vi "Sort into Arrival Time Buffer.vi"(5 "Time Low":u32[][](array[numeric]), 6 "Delay, ns":u32, 7 "Time High":u32[][](array[numeric]), 8 "Channel buffers are synchronized":bool, 9 "Size of Channel Arrays":u32[](array[numeric]), 10 "Buffer In":i32[][](array[numeric]), 11 "Number of Photons Counted In":i32) -> (1 "Index for Buffer":i32[](array[numeric]), 2 "Buffer Out":i32[][](array[numeric]), 3 "Number of Photons Counted Out":i32)   [LabVIEW 2009]
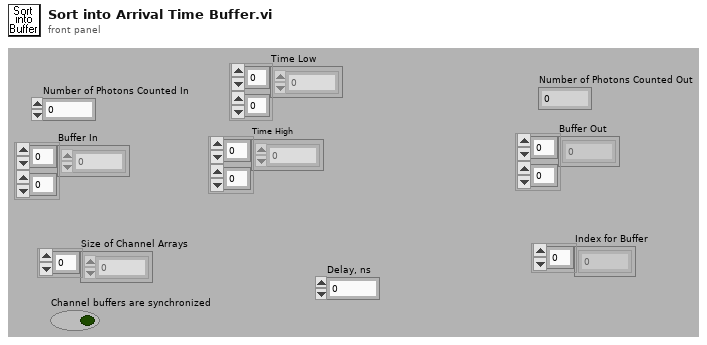
[diagram p1: front panel]
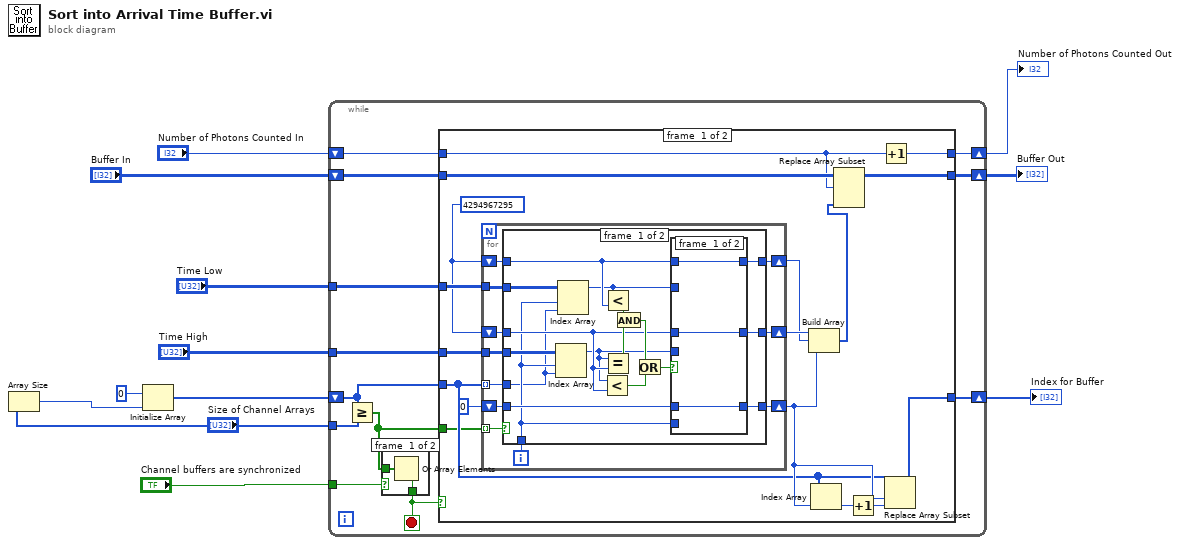
[diagram p0: block diagram]
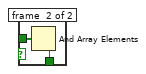
[diagram p2: hidden frame]
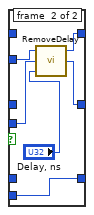
[diagram p3: hidden frame]
diagram:
  n1 = Array Size(array="Size of Channel Arrays") -> (size(s)=w1:i32)
  n2 = Initialize Array(0 ("Element Data"), w1) -> (w5:i32[])
  n3 = while {
    tunnel: "Channel buffers are synchronized" -> [w13]
    shift-left: "Number of Photons Counted In" -> [w18]
    shift-right: [w17] -> w12
    shift-left: "Buffer In" -> [w22]
    shift-right: [w19] -> w8
    shift-left: w5 -> [w23]
    shift-right: [w16] -> w10
    tunnel: "Size of Channel Arrays" -> [w24]
    tunnel: "Time High" -> [w20]
    tunnel: "Time Low" -> [w21]
    stop <- w14 stop-if-true
    n4 = Greater Or Equal?(x=w23, y=w24) -> (x >= y?=w15:bool[])
    n5 = case shown="True" w13 {
      tunnel: [w26 w27] -> w14
      tunnel: w15 -> [w25 w28]
      frame #0 {
        n6 = Or Array Elements(Boolean array=w25) -> (logical OR=w26:bool)
      }
      frame #1 {
        n7 = And Array Elements(Boolean array=w28) -> (logical AND=w27:bool)
      }
    }
    n8 = case shown="False" w14 {
      tunnel: w23 -> [w32 w86]
      tunnel: w22 -> [w41 w88]
      tunnel: w21 -> [w45 _]
      tunnel: w20 -> [w44 _]
      tunnel: [w40 w88] -> w19
      tunnel: [w38 w87] -> w17
      tunnel: w18 -> [w39 w87]
      tunnel: [w31 w86] -> w16
      tunnel: w15 -> [w30 _]
      frame #0 {
        w43 = u32 4294967295
        n9 = for {
          tunnel: w45 -> [w56]
          tunnel: w44 -> [w55]
          tunnel: w32 -> [w53] mode=indexing
          shift-right: [w49] -> w36
          shift-left: w43 -> [w51]
          shift-right: [w48] -> w37
          shift-left: w43 -> [w52]
          shift-right: [w47] -> w33
          shift-left: 0 -> [w50]
          tunnel: w30 -> [w46] mode=indexing
          i -> [w54]
          n10 = case shown="False" w46 {
            tunnel: w56 -> [w62 _]
            tunnel: w55 -> [w60 _]
            tunnel: w54 -> [w59 _]
            tunnel: w53 -> [w58 _]
            tunnel: w52 -> [w68 w84]
            tunnel: w51 -> [w67 w85]
            tunnel: w50 -> [w66 w83]
            tunnel: [w65 w85] -> w49
            tunnel: [w64 w84] -> w48
            tunnel: [w63 w83] -> w47
            frame #0 {
              n11 = Index Array(array=w60, index (row)=w59, index (col)=w58) -> (element=w57:u32)
              n12 = Index Array(array=w62, index (row)=w59, index (col)=w58) -> (element=w61:u32)
              n13 = Less?(x=w57, y=w68) -> (x < y?=w71:bool)
              n14 = Less?(x=w61, y=w67) -> (x < y?=w73:bool)
              n15 = Equal?(x=w57, y=w68) -> (x = y?=w72:bool)
              n16 = And(x=w73, y=w72) -> (x .and. y?=w70:bool)
              n17 = Or(x=w70, y=w71) -> (x .or. y?=w69:bool)
              n18 = case shown="True" w69 {
                tunnel: w68 -> [w75 _]
                tunnel: w67 -> [w76 _]
                tunnel: w66 -> [w74 _]
                tunnel: w61 -> [_ w81]
                tunnel: w57 -> [_ w80]
                tunnel: w59 -> [_ w82]
                tunnel: [w76 w78] -> w65
                tunnel: [w75 w77] -> w64
                tunnel: [w74 w82] -> w63
                frame #0 {
                }
                frame #1 {
                  n19 = call "RemoveDelay.vi"("Delay, ns"="Delay, ns", "Time High"=w80, "Time Low"=w81) -> ("Time High New"=w77:u32, "Time Low New"=w78:u32)  [unwired: 1 in]
                }
              }
            }
            frame #1 {
            }
          }
        }
        n20 = Build Array(w37, w36, w33) -> (w29:u32[])
        n21 = Index Array(array=w32, index=w33) -> (element=w35:i32)
        n22 = Replace Array Subset(array=w41, new element=w29, index (row)=w39) -> (w40:i32[][])  [unwired: 1 in]
        n23 = Increment(x=w35) -> (x+1=w34:i32)
        n24 = Increment(x=w39) -> (x+1=w38:i32)
        n25 = Replace Array Subset(array=w32, new element=w34, index=w33) -> (w31:i32[])
      }
      frame #1 {
      }
    }
  }
  "Number of Photons Counted Out" <- w12
  "Buffer Out" <- w8
  "Index for Buffer" <- w10
